vi "Validate User Input.vi"(8 "error in (no error)":errorcluster, 9 "available measurement names":string[](array[string]), 10 "project ref":refnum<vi>, 11 "multicolumnListbox in":refnum<vi>) -> (0 "error out":errorcluster, 2 "warning?":bool, 3 "multicolumnListbox out":refnum<vi>)   [LabVIEW 2021, in "MeasurementClient Editor.lvlib"]
uses:
  MeasurementClient Editor.lvlib
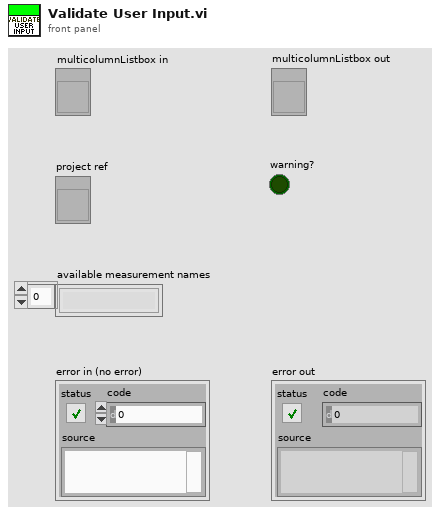
[diagram p1: front panel]
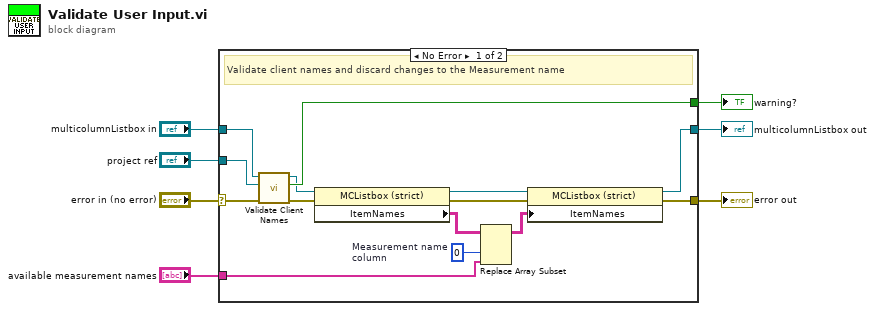
[diagram p0: block diagram]
diagram:
  n1 = case shown="No Error" "error in (no error)" {
    selector: "error in (no error)" -> [w20 w22]
    tunnel: "multicolumnListbox in" -> [w21 w23]
    tunnel: "project ref" -> [w18 _]
    tunnel: [w17 _] -> w4
    tunnel: "available measurement names" -> [w12 _]
    tunnel: [w11 w22] -> w2
    tunnel: [w8 w23] -> w1
    frame No Error {
      w13 = 0  # Measurement name column
      # "Validate client names and discard changes to the Measurement name"
      n2 = call "Validate Client Names.vi"("error in (no error)"=w20, "project ref"=w18, "multicolumnListbox in"=w21) -> ("error out"=w19:errorcluster, "warning?"=w17:bool, "multicolumnListbox out"=w15:refnum<vi>)  [unwired: 6 in]
      n3 = property class="MCListbox (strict)"(reference=w15, error in=w19) -> (reference out=w10:refnum<vi>, error out=w16:errorcluster, "ItemNames"=w14:string[][])
      n4 = Replace Array Subset(array=w14, new element=w12, index (col)=w13) -> (w9:string[][])  [unwired: 1 in]
      n5 = property class="MCListbox (strict)"(reference=w10, error in=w16, "ItemNames"=w9) -> (reference out=w8:refnum<vi>, error out=w11:errorcluster)
    }
    frame Error {
      # "Pass"
    }
  }
  "error out" <- w2
  "multicolumnListbox out" <- w1
  "warning?" <- w4
